vi "Read Instrument.vi"(8 "error in (no error)":errorcluster, 11 "VISA resource name":refnum<visa-resource-name>="GPIB12::28::INSTR") -> (0 "error out":errorcluster, 2 "Measurement":T1, 3 "VISA resource name out":refnum<visa-resource-name>)   [LabVIEW 2019, in "AH2500A.lvclass"]
uses:
  AH2500A.lvclass
  Typedefs/AH2500A Measurement--Cluster.ctl
panel:
  out "read buffer":string
  # "Do a single measurement"
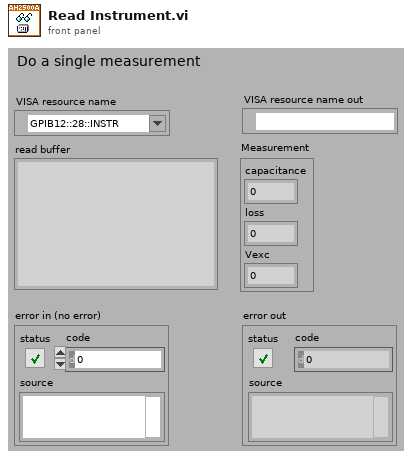
[diagram p1: front panel]
types:
  T1 = typedef "AH2500A.lvclass/AH2500A Measurement--Cluster.ctl" = cluster{"capacitance":dbl, "loss":dbl, "Vexc":dbl}
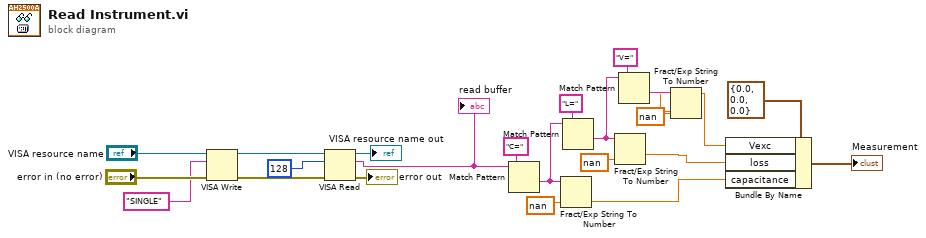
[diagram p0: block diagram]
diagram:
  n1 = VISA Write(VISA resource name="VISA resource name", write buffer="SINGLE", error in (no error)="error in (no error)") -> (VISA resource name out=w22:refnum<visa-resource-name>, error out=w21:errorcluster)  [unwired: 1 out]
  n2 = VISA Read(VISA resource name=w22, byte count=u32 128, error in (no error)=w21) -> (VISA resource name out=→"VISA resource name out":refnum<visa-resource-name>, read buffer=w1:string, error out=→"error out":errorcluster)  [unwired: 1 out]
  "read buffer" <- w1
  n3 = Match Pattern(string=w1, regular expression="C=") -> (after substring=w16:string)  [unwired: 1 in, 3 out]
  n4 = Fract/Exp String To Number(string=w16, default (0 dbl)=nan) -> (number=w9:dbl)  [unwired: 2 in, 1 out]
  n5 = Match Pattern(string=w16, regular expression="L=") -> (after substring=w11:string)  [unwired: 1 in, 3 out]
  n6 = Fract/Exp String To Number(string=w11, default (0 dbl)=nan) -> (number=w8:dbl)  [unwired: 2 in, 1 out]
  n7 = Match Pattern(string=w11, regular expression="V=") -> (after substring=w14:string)  [unwired: 1 in, 3 out]
  n8 = Fract/Exp String To Number(string=w14, default (0 dbl)=nan) -> (number=w7:dbl)  [unwired: 2 in, 1 out]
  n9 = Bundle By Name(cluster=T1 {"capacitance"=0.0, "loss"=0.0, "Vexc"=0.0} ("Measurement"), "Vexc"=w7, "loss"=w8, "capacitance"=w9) -> (→"Measurement":T1)
